vi "Test Snake Initial Position.vi"(8 "error in (no error)":errorcluster, 11 "Test Case In":refnum<class "Snake Test.lvclass">) -> (0 "error out":errorcluster, 3 "Test Case Out":refnum<class "Snake Test.lvclass">)   [LabVIEW 2020, in "Snake Test.lvclass"]
uses:
  Snake Test.lvclass
  Snake Test.lvclass/Snake Test.ctl
  source/Snake/Snake.lvclass
  source/Particle/Position.ctl
  source/Particle.lvclass
  <vilib>/Astemes/LUnit/Test Case.lvclass
  C:/Program Files (x86)/National Instruments/LabVIEW 2020/vi.lib/Astemes/LUnit/Test Case.lvclass
  C:/git/astemes-snake-game/tests/Snake Test/Snake Test.lvclass
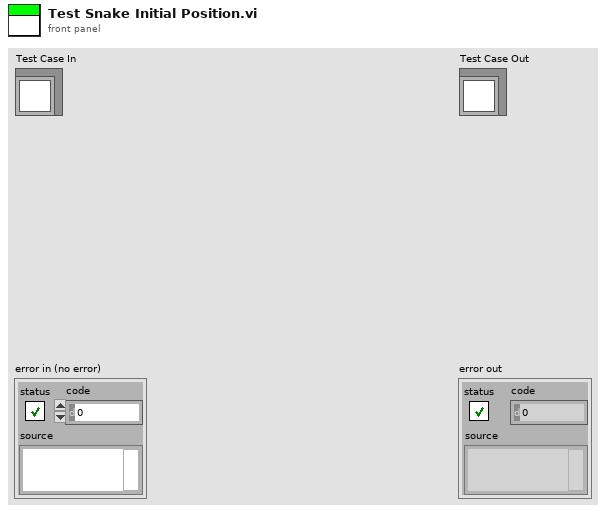
[diagram p1: front panel]
types:
  T1 = typedef "Particle.lvclass/Position.ctl" = cluster{"X":i32, "Y":i32}
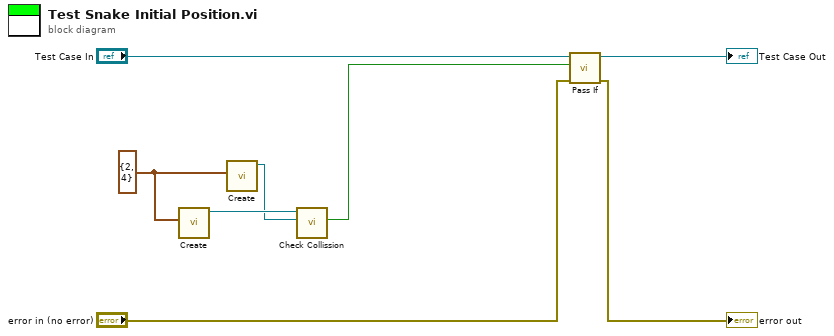
[diagram p0: block diagram]
diagram:
  w3 = T1 {"X"=2, "Y"=4} ("Position")
  n1 = call "Create.vi"("Position"=w3) -> ("Snake out"=w4:refnum<class "Snake.lvclass">)  [unwired: 10 in]
  n2 = call "Create.vi"("Position"=w3) -> ("Particle out"=w2:refnum<class "Particle.lvclass">)  [unwired: 10 in]
  n3 = call "Check Collission.vi"("Particle"=w2, "Snake in"=w4) -> ("Collided?"=w1:bool)  [unwired: 8 in, 1 out]
  n4 = call <vilib>:"Pass If.vi"("error in (no error)"="error in (no error)", "Pass?"=w1, "LUnit Test Case In"="Test Case In") -> ("error out"=→"error out":errorcluster, "LUnit Test Case Out"=→"Test Case Out":refnum<class "Snake Test.lvclass">)  [unwired: 7 in]
